vi "Abort Sequence text out.vi"() -> (0 "Command text":string[][](array[string]))   [LabVIEW 2020]
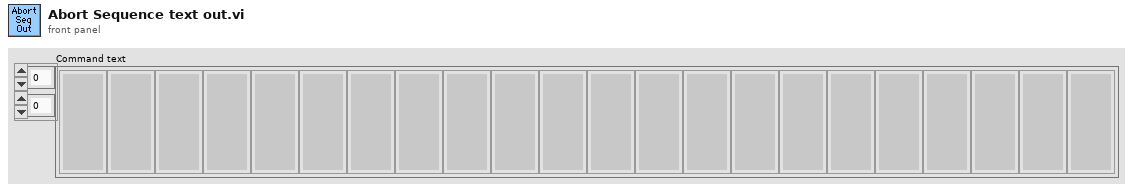
[diagram p1: front panel]
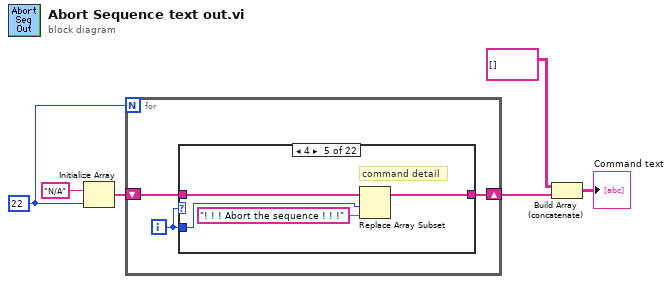
[diagram p0: block diagram]
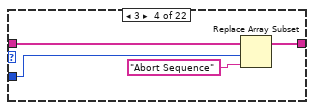
[diagram p5: hidden frame]
diagram:
  w1 = 22
  n1 = Initialize Array("N/A", w1) -> (w2:string[])
  n2 = for {
    N: w1 -> [_]
    shift-right: [w7] -> w4
    shift-left: w2 -> [w8]
    i -> [w9]
    n3 = case shown="4" w9 {
      tunnel: w9 -> [_ _ _ w14 w20 _ _ _ _ _ _ _ _ _ _ _ _ _ _ _ _ _]
      tunnel: w8 -> [w10 w11 w12 w16 w18 w21 w22 w23 w24 w25 w26 w27 w28 w29 w30 w31 w32 w33 w34 w35 w36 w37]
      tunnel: [w10 w11 w12 w15 w19 w21 w22 w23 w24 w25 w26 w27 w28 w29 w30 w31 w32 w33 w34 w35 w36 w37] -> w7
      frame 0, Default {
        # "Line #"
      }
      frame 1 {
      }
      frame 2 {
        # "instrument address"
      }
      frame 3 {
        n4 = Replace Array Subset(array=w16, new element="Abort Sequence" ("new element/subarray"), index=w14) -> (w15:string[])
      }
      frame 4 {
        # "command detail"
        n5 = Replace Array Subset(array=w18, new element="! ! ! Abort the sequence ! ! !" ("new element/subarray"), index=w20) -> (w19:string[])
      }
      frame 5 {
        # "in  case 1"
      }
      frame 6 {
        # "in case 2"
      }
      frame 7 {
      }
      frame 8 {
      }
      frame 9 {
      }
      frame 10 {
      }
      frame 11 {
      }
      frame 12 {
      }
      frame 13 {
      }
      frame 14 {
      }
      frame 15 {
      }
      frame 16 {
      }
      frame 17 {
      }
      frame 18 {
      }
      frame 19 {
      }
      frame 20 {
      }
      frame 21 {
      }
    }
  }
  n6 = Build Array (concatenate)(string[][] [], w4) -> (→"Command text":string[][])
